vi "Add Item Buffered.vi"(7 "Items Array Length":i32=5, 8 "错误输入":errorcluster, 10 "Item":string, 11 "Listbox Ref":refnum<vi>) -> (0 "错误输出":errorcluster, 3 "Dup Listbox Ref":refnum<vi>)   [LabVIEW 2012, in "Listbox Tool.lvlib"]
uses:
  Listbox Tool.lvlib
  Custom Type/Read and Write Mode.ctl
  Property/Set and Get ItemNames.vi
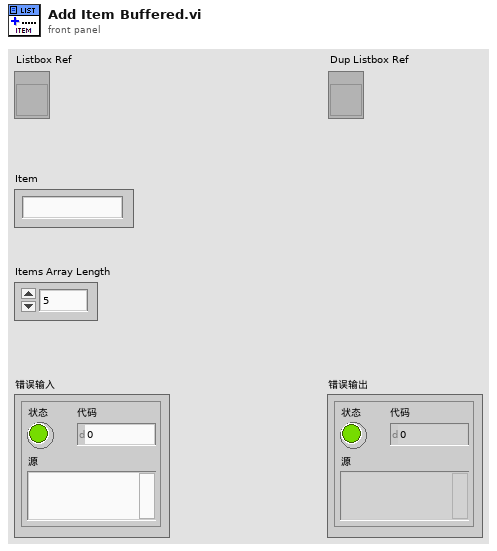
[diagram p1: front panel]
types:
  T1 = typedef "Listbox Tool.lvlib/Read and Write Mode.ctl" = enum16{"Read", "Write"}
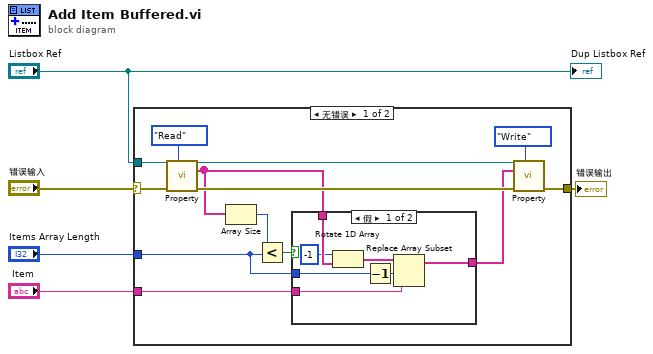
[diagram p0: block diagram]
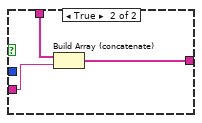
[diagram p2: hidden frame]
diagram:
  n1 = case shown="无错误" "错误输入" {
    selector: "错误输入" -> [w18 w29]
    tunnel: "Listbox Ref" -> [w17 _]
    tunnel: "Item" -> [w9 _]
    tunnel: [w13 w29] -> w2
    tunnel: "Items Array Length" -> [w7 _]
    frame No Error {
      n2 = call-poly "Property.vi"("Mode"=Read_and_Write_Mode."Read", "错误输入"=w18, "Listbox Ref"=w17) -> ("错误输出"=w16:errorcluster, "ItemNames Out"=w10:string[], "Dup Listbox Ref"=w15:refnum<vi>)  [unwired: 6 in]
      n3 = Array Size(array=w10) -> (size(s)=w12:i32)
      n4 = Less?(x=w12, y=w7) -> (x < y?=w11:bool)
      n5 = case shown="假" w11 {
        tunnel: w10 -> [w25 w28]
        tunnel: w9 -> [w22 w27]
        tunnel: [w21 w26] -> w8
        tunnel: w7 -> [w19 _]
        frame False {
          n6 = Rotate 1D Array(1:w25, 2:-1 ("n")) -> (0:w23:string[])
          n7 = Decrement(x=w19) -> (x-1=w20:i32)
          n8 = Replace Array Subset(array=w23, new element=w22, index=w20) -> (w21:string[])
        }
        frame True {
          n9 = Build Array (concatenate)(w28, w27) -> (w26:string[])
        }
      }
      n10 = call-poly "Property.vi"("Mode"=Read_and_Write_Mode."Write", "错误输入"=w16, "ItemNames In"=w8, "Listbox Ref"=w15) -> ("错误输出"=w13:errorcluster)  [unwired: 5 in, 2 out]
    }
    frame Error {
    }
  }
  "错误输出" <- w2
  "Dup Listbox Ref" <- "Listbox Ref"
